vi "host_get_target.vi"(8 "error in":errorcluster) -> (0 "error out":errorcluster, 3 "target":T1)   [LabVIEW 2021]
doc: "Get current target on the FPGA."
uses:
  fpga/fpga_dtype_sgl_8ch.ctl
  core/host_global_vars.vi
  <vilib>/Utility/error.llb/Error Cluster From Error Code.vi
  <vilib>/rvi/errors/niLvFpgaAdjustHostInterfaceError.vi
  <vilib>/rvi/interface/nirviReadWriteControl/nirviReadWriteControl.xnode
  FPGA Bitfiles/openlabspm_FPGATarget_fpgamain_eo-gUZR5D1g.lvbitx
  fpga/fpga_main.vi
  NiFpgaLv.dll
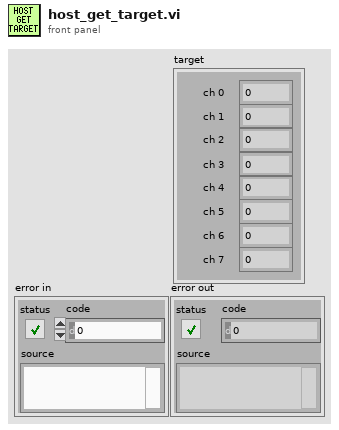
[diagram p1: front panel]
types:
  T1 = typedef "fpga_dtype_sgl_8ch.ctl" = cluster{"ch 0":sgl, "ch 1":sgl, "ch 2":sgl, "ch 3":sgl, "ch 4":sgl, "ch 5":sgl, "ch 6":sgl, "ch 7":sgl}
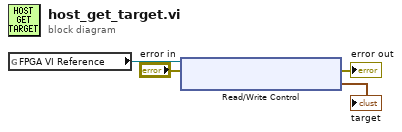
[diagram p0: block diagram]
diagram:
  n1 = global read "host_global_vars.vi" "FPGA VI Reference"() -> (w4:refnum<k20>)
  n2 = xnode "Read/Write Control"("FPGA VI Reference In"=w4, "error in"="error in") -> ("error out"=→"error out":errorcluster, "target"=→"target":T1)  [unwired: 1 out]
